vi "i2c_mux_demux.vi"() -> ()   [LabVIEW 2014]
uses:
  mux_state.ctl
  demux_state.ctl
  Common/fractional_phase.ctl
  <vilib>/Platform/TimedLoop/XDataNode/timing_clust.ctl
  <vilib>/Platform/TimedLoop/XDataNode/nitl_modes.ctl
  <vilib>/Platform/TimedLoop/XDataNode/wakeup.ctl
  Common/i2c_status.ctl
  Common/demux_command.ctl
  Common/i2c_command.ctl
  <vilib>/rvi/Emulation/niFpgaGetClockAttributes.vi
  <vilib>/rvi/Emulation/niFpgaSctlEmulationGetInTimedLoop.vi
  <vilib>/rvi/Emulation/niFpgaEmulationReportErrorSimple.vi
  <vilib>/rvi/DataTransferAndStorage/Container/Common/niFpgaContainerExecOnDevCompGetState.vi
  <vilib>/rvi/Emulation/niFpgaEmulationIsFPGAContextNoSignature.vi
  <vilib>/rvi/errors/niFpgaSetErrorForExecOnDevCompSimple.vi
  <vilib>/rvi/eio/common/nirviEmuReportErrorAndStop.vi
  <vilib>/rvi/DataTransferAndStorage/Container/Common/niFpgaContainerGetUniqueNameForEmu.vi
  <vilib>/rvi/FIFO/Fifo_Resource/nirvififoEmulationSetSize.vi
  <vilib>/rvi/FIFO/Fifo_Resource/nirviFifoEmulationQueueMgr.vi
  <instcachedir>/0/nirviFifoEmulationQueueMgr_E5CAEC123FF24DC58D834DCA3CDAA9B5.lvgen/nirviFifoEmulationQueueMgr_E5CAEC123FF24DC58D834DCA3CDAA9B5_002.vi
  <vilib>/rvi/FIFO/Fifo_Resource/nirvififoEmulationDetermineInputValidOut.vi
  <vilib>/rvi/FIFO/Fifo_Resource/nirvififoEmulationCreateLock.vi
  <vilib>/rvi/Emulation/niFpgaProcessEmulError.vi
  <vilib>/rvi/FIFO/Fifo_Resource/nirvififoEmulationObtainLock.vi
  <vilib>/rvi/FIFO/Fifo_Resource/nirvififoEmulationReleaseLock.vi
  <vilib>/rvi/occurrence/nirviWaitOnOccurrenceBase.vi
  <vilib>/rvi/errors/nirviReportUnexpectedCaseInternalError.vi
  <vilib>/rvi/errors/nirviReportUnexpectedCaseInternalError (U32).vi
  <vilib>/Utility/error.llb/Clear Errors.vi
  <vilib>/rvi/interface/RandomDataEmulation/niFpgaRandomDataHandleErrors.vi
  <vilib>/rvi/Emulation/niFpgaCriticalErrorInLSC.vi
  <instcachedir>/0/nirviFifoEmulationQueueMgr_E5CAEC123FF24DC58D834DCA3CDAA9B5.lvgen/nirviFifoEmulationQueueMgr_E5CAEC123FF24DC58D834DCA3CDAA9B5_001.vi
  <vilib>/rvi/eio/common/nirviEmuTemplateMethod_errors.vi
  <vilib>/rvi/DataTransferAndStorage/Container/XNode/niFpgaContainer.xnode
  <vilib>/rvi/FIFO/Fifo_Resource/niFpgaFifoEmulationRefIn.vi
  <vilib>/Platform/TimedLoop/XDataNode/XDataNode.xnode
  <vilib>/eio/EIONode/EIONode.xnode
  <vilib>/Platform/TimedLoop/XDataNode/XDNodeRunTimeDep.lvlib
  fpga_globals.vi
panel:
  in  "Lo rate half period":u16
  out "FPGA code version":i16
  in  "ASAP timer phase advance":T1[](array[typedef])=[0.0, 0.0, 0.0, 0.0, 0.0, 0.0]
  out "Sequence num":u8
  in  "Command hard trigger":bool=TRUE
  in  "Output enable":bool[](array[boolean])=[FALSE, FALSE, FALSE, FALSE, FALSE, FALSE]
  out "Drain count":u8
  out "Hard trigger mode":bool
  out "Drain FIFO":bool
  out "Demux data":u8
  out "Demux  Read inhibit":bool
  out "Hardware trigger enable":bool
  in  "Finder":bool
  in  "ASAP timer initial phase":T1[](array[typedef])=[0.0, 0.0, 0.0, 0.0, 0.0, 0.0]
  out "Timestamp":u16
  out "Trigger wait":bool
  out "Local FIFO full":bool
  out "Demux bus number":fxp<+,8,8>
  out "Demux data ready":bool
  out "Demux state":T2
  out "Mux bus number":fxp<+,3,3>
  out "Host FIFO full":bool
  out "Mux Read inhibit":bool
  out "Mux data ready":bool
  out "Mux data":u8
  out "Mux state":T3
  in  "I2C clock divisor":u8=25
  # "Current timestamp\nfor I2C status notifications."
  # "ASAP finder switch"
  # "The phase in radians is pi times this number. See phase_timer_out.vi for details"
  # "Enable timer outputs"
  # "If true, command operation uses hard trigger mode,\notherwise soft trigger."
  # "Locals:"
  # "Debugging:"
  # "Command sequence number, from host command FIFO"
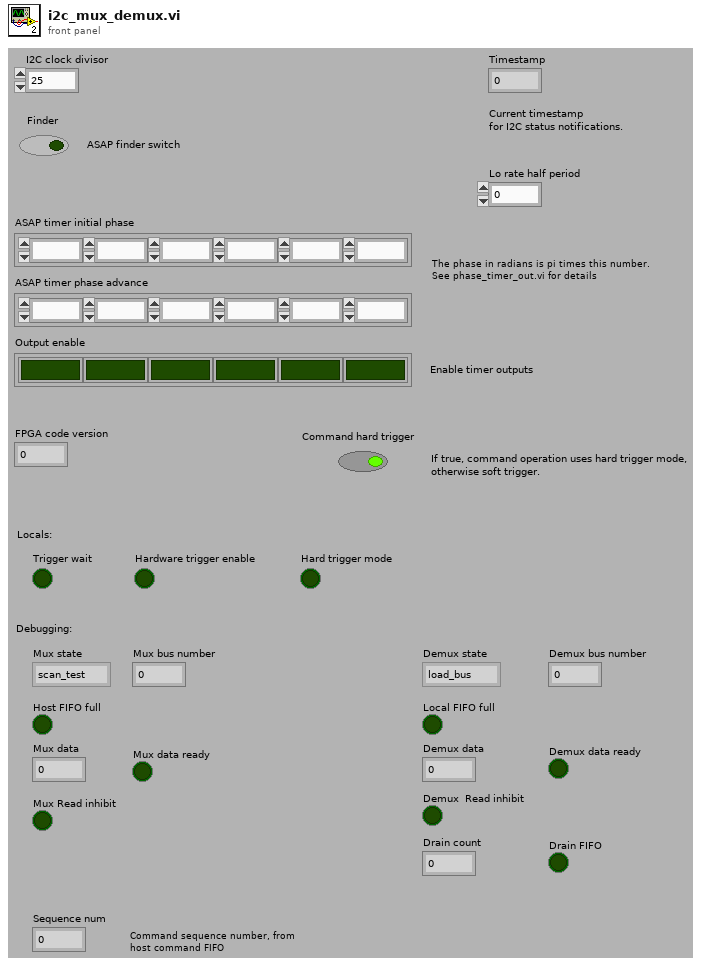
[diagram p1: front panel]
types:
  T1 = typedef "fractional_phase.ctl" = fxp<+,32,1>
  T2 = typedef "demux_state.ctl" = enum8{"load_bus", "load_count", "copying", "wait_trigger"}
  T3 = typedef "mux_state.ctl" = enum8{"scan_test", "push_bus", "push_TS_hi", "push_TS_lo", "copy_code", "load_arg", "copy_arg", "load_count", "copy_data"}
  T4 = typedef "XDNodeRunTimeDep.lvlib/timing_clust.ctl" = cluster{"Expected End [f-1]":u64, "Actual End [f-1]":u64, "Finished Late? [f-1]":bool, "Expected End [i-1]":u64, "Actual End [i-1]":u64, "Finished Late? [i-1]":bool, "Expected Start [i]":u64, "Actual Start [i]":u64, "Expected Start [f]":u64, "Actual Start [f]":u64, "Source Name":string, "Structure Name":string, "Period":i64, "Deadline":i64, "Offset":i64, "Start":i64, "Priority":i32, "Timeout":i32, "Mode":T5, "Wakeup Reason":T6, "Error":errorcluster, "Source Type":string, "Secondary Source Type":string, "Global End Time":u64, "Global Start Time":u64, "Frame Duration":u64, "Iteration Duration":u64, "Assigned CPU":i32, "I/O Scan Engine Mode":u32}
  T5 = typedef "XDNodeRunTimeDep.lvlib/nitl_modes.ctl" = enum32{"No Change", "Process missed periods, maintain original phase", "Discard missed periods, maintain original phase", "Process missed periods, ignore original phase", "Discard missed periods, ignore original phase"}
  T6 = typedef "XDNodeRunTimeDep.lvlib/wakeup.ctl" = enum32{"Normal", "Aborted", "Asynchronous wakeup", "Timing source error", "Timed loop error", "Timeout"}
  T7 = typedef "i2c_status.ctl" = enum8{"Invalid", "Command", "I2C start", "Trigger wait", "TX data wait", "Sequence", "Receive data", "I2C error", "Address NACK", "Data NACK", "SDA stuck", "SCL stuck", "Bad command"}
  T8 = typedef "demux_command.ctl" = enum8{"bus_0", "bus_1", "bus_2", "invalid_3", "invalid_4", "drain_fifo", "wait_hard_trigger", "wait_soft_trigger", "trigger_enable"}
  T9 = typedef "i2c_command.ctl" = enum8{"invalid", "start_write", "start_read", "stop", "sequence"}
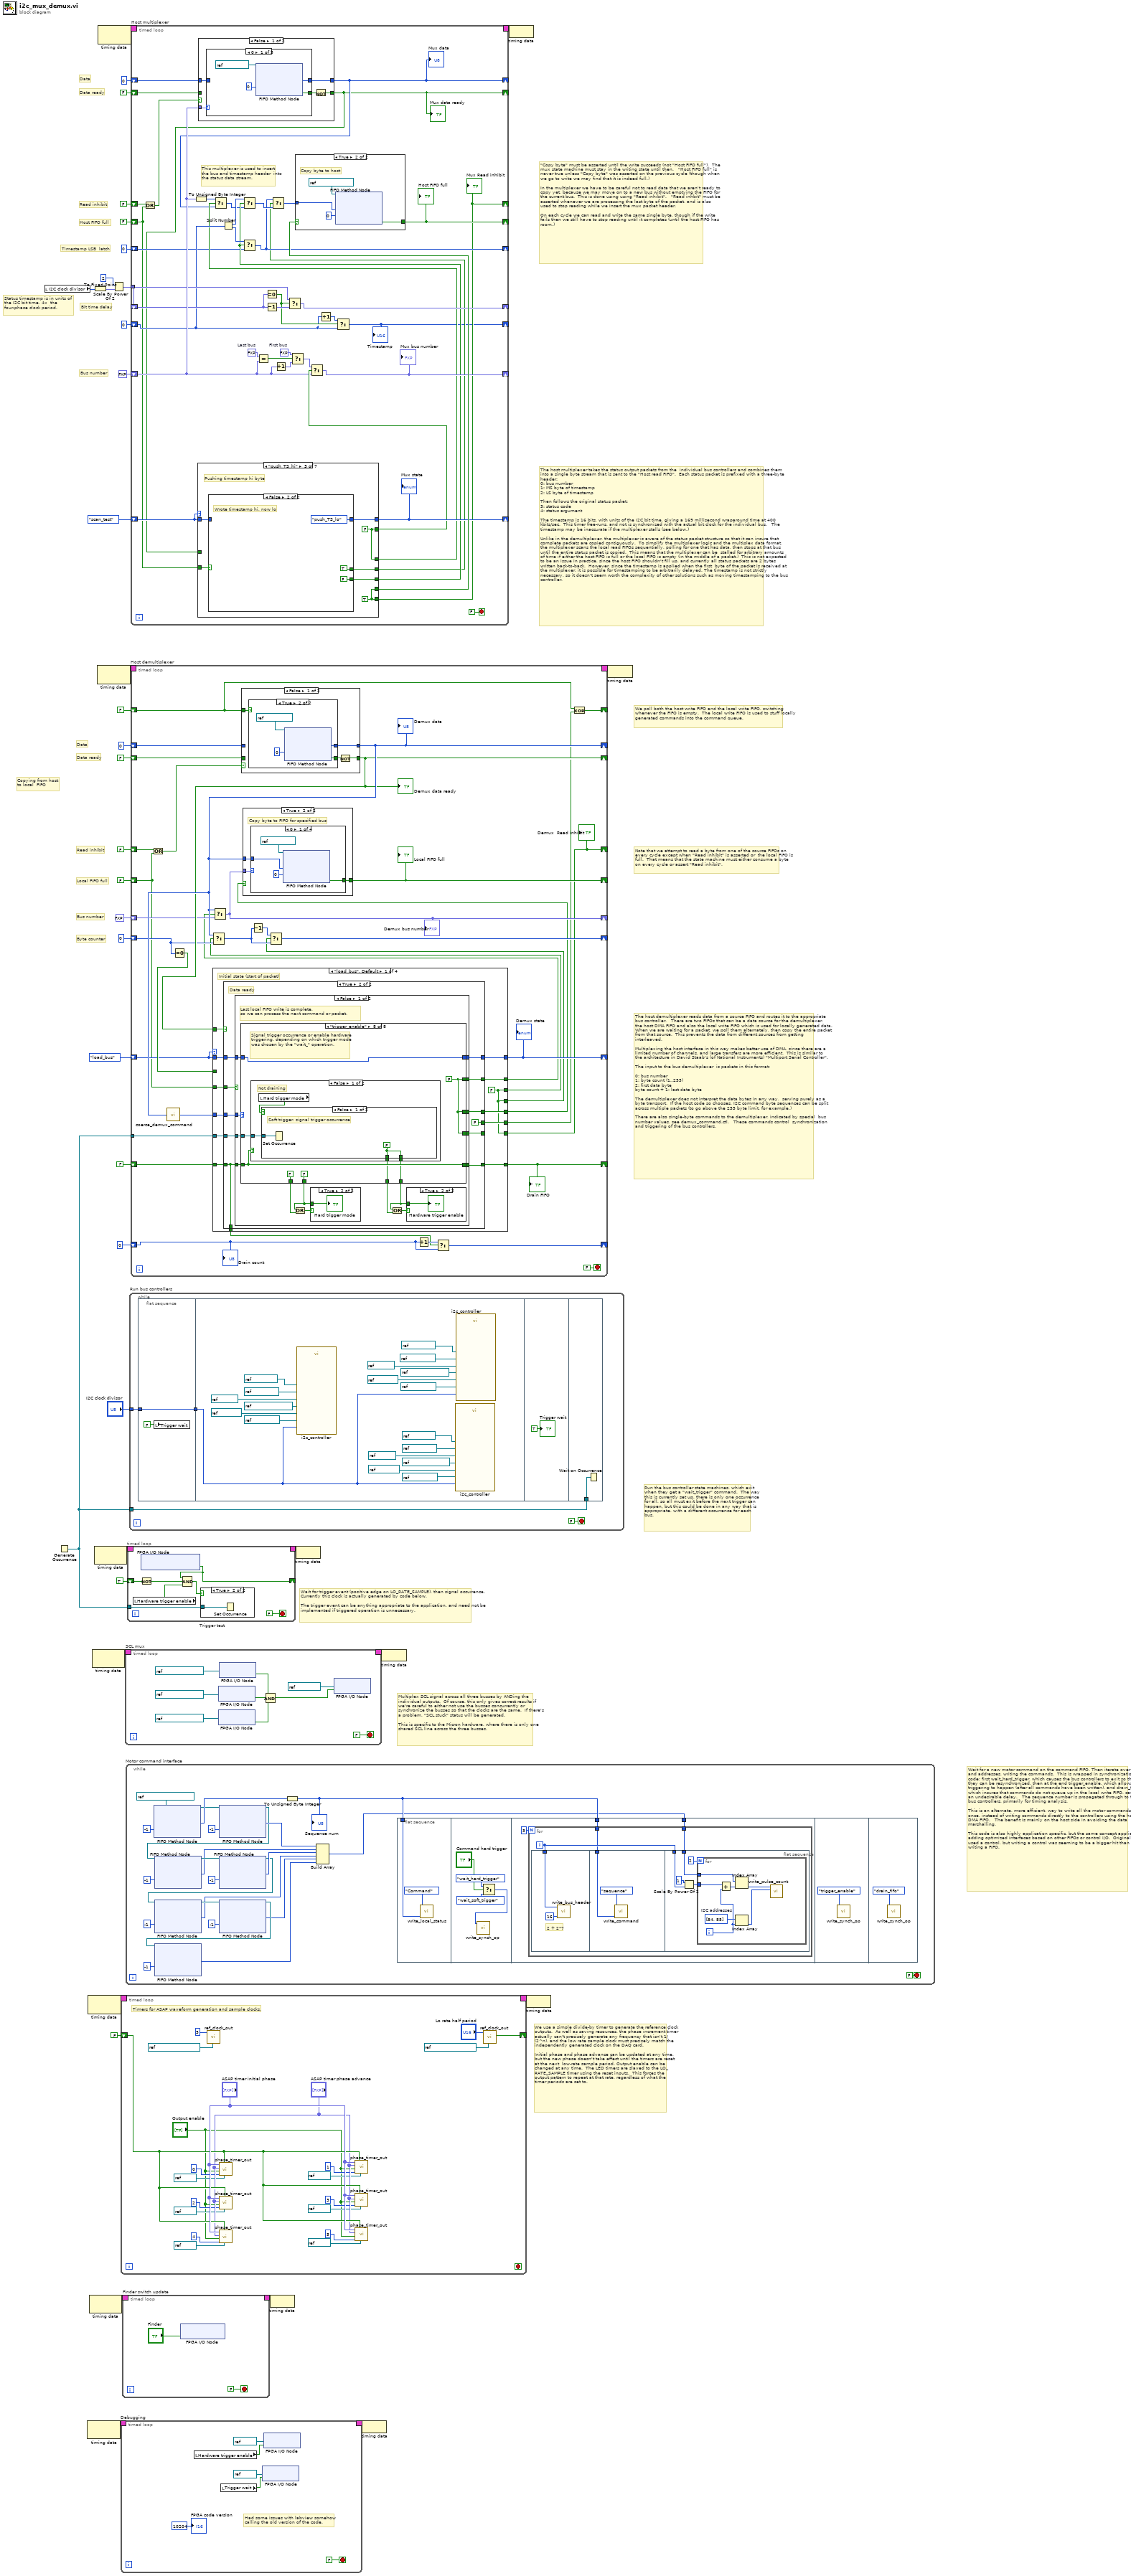
[diagram p0: block diagram]
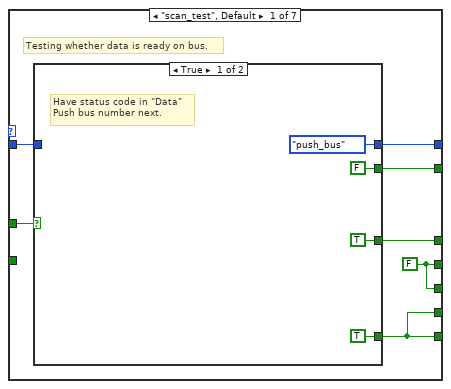
[diagram p3: hidden frame]
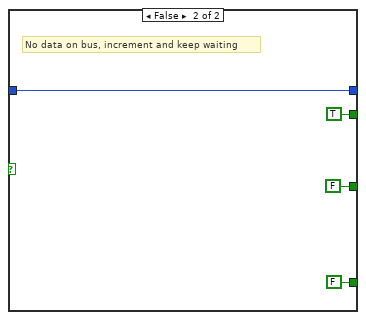
[diagram p4: hidden frame]
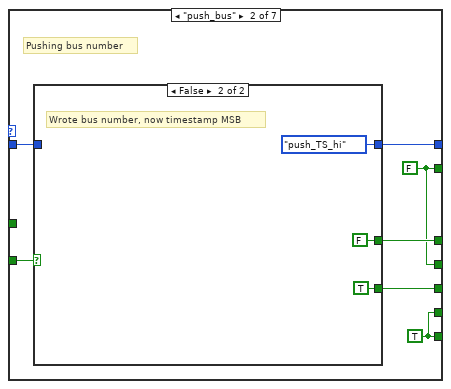
[diagram p5: hidden frame]
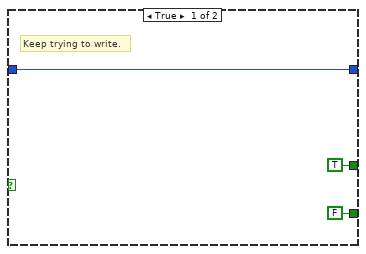
[diagram p6: hidden frame]
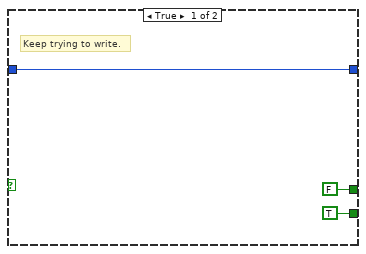
[diagram p7: hidden frame]
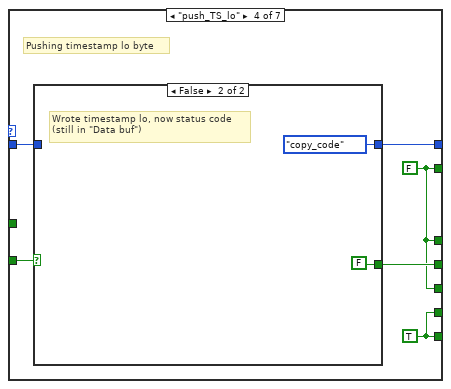
[diagram p8: hidden frame]
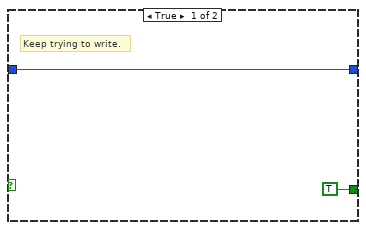
[diagram p9: hidden frame]
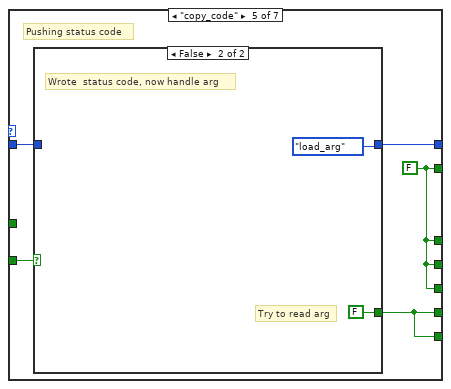
[diagram p10: hidden frame]
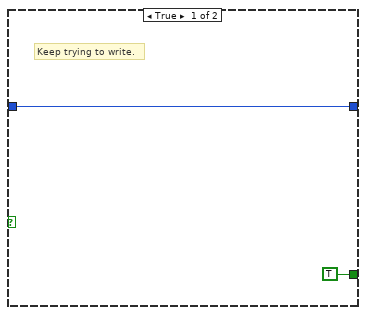
[diagram p11: hidden frame]
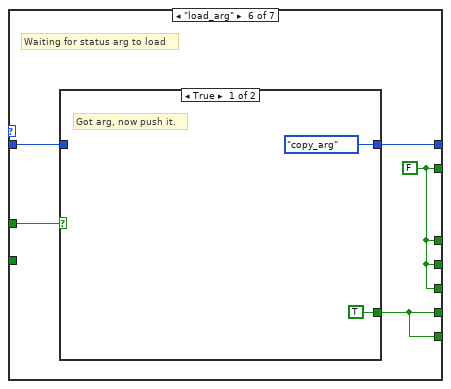
[diagram p12: hidden frame]
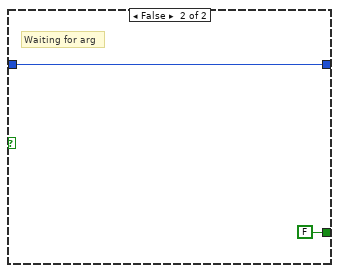
[diagram p13: hidden frame]
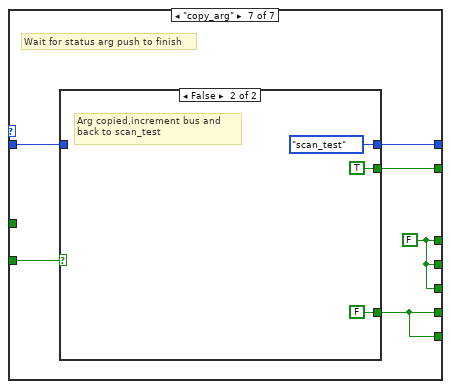
[diagram p14: hidden frame]
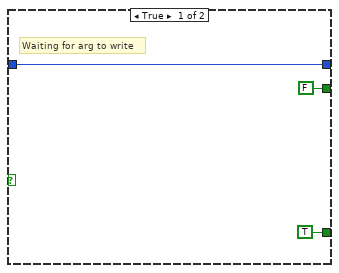
[diagram p15: hidden frame]
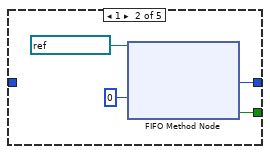
[diagram p16: hidden frame]
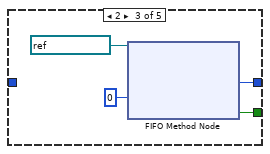
[diagram p17: hidden frame]
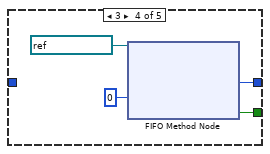
[diagram p18: hidden frame]
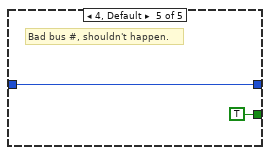
[diagram p19: hidden frame]
diagram:
  # "We use a simple divide-by timer to generate the reference clock outputs.  As well as saving resources, the phase increment timer actually can't precisely generate any frequency that isn't 1/(2^n), and the low rate sample clock must precisely match the independently generated clock on the DAQ card.\n\nInitial phase and phase advance can be updated at any time, but the new phase doesn't take effect until the timers are reset at the next  low-rate sample period. Output enable can be changed at any time.  The LED timers are slaved to the LO_RATE_SAMPLE timer using the reset inputs.  This forces the output pattern to repeat at that rate, regardless of what the timer periods are set to."
  # "Read inhibit"
  # "We poll both the host write FIFO and the local write FIFO, switching whenever the FIFO is empty.  The local write FIFO is used to stuff locally generated commands into the command queue."
  # "Multiplex SCL signal across all three busses by ANDing the individual outputs.  Of course, this only gives correct results if we're careful to either not use the busses concurrently or synchronize the busses so that the clocks are the same.  If there's a problem, \"SCL stuck\" status will be generated.\n\nThis is specific to the Micron hardware, where there is only one shared SCL line across the three busses."
  # "Wait for a new motor command on the command FIFO. Then iterate over buses and addresses, writing the commands.  This is wrapped in synchronization code: first wait_hard_trigger, which causes the bus controllers to exit so that they can be resynchronized, then at the end trigger_enable, which allows triggering to happen (after all commands have been written), and drain_fifo, which insures that commands do not queue up in the local write FIFO, causing an undesirable delay.   The sequence number is propagated through to the bus controllers, primarily for timing analysis.\n\nThis is an alternate, more efficient, way to write all the motor commands at once, instead of writing commands directly to the controllers using the host DMA FIFO.   The benefit is mainly on the host side in avoiding the data marshalling.\n\nThis code is also highly application specific, but the same concept applies of adding optimized interfaces based on other FIFOs or control I/O.  Originally this used a control, but writing a control was seeming to be a bigger hit than writing a FIFO."
  # "Run the bus controller state machines, which exit when they get a \"wait_trigger\" command.  The way this is currently set up, there is only one occurrence for all, so all must exit before the next trigger can happen, but this could be done in any way that is appropriate, with a different occurrence for each bus."
  # "Wait for trigger event (positive edge on LO_RATE_SAMPLE), then signal occurrence.  Currently this clock is actually generated by code below.\n\nThe trigger event can be anything appropriate to the application, and need not be implemented if triggered operation is unnecessary."
  # "\"Copy byte\" must be asserted until the write succeeds (not \"Host FIFO full\").  The mux state machine must stay in the writing state until then.   \"Host FIFO full\" is never true unless \"Copy byte\" was asserted on the previous cycle (though when we go to write we may find that it is indeed full.)\n\nIn the multiplexer we have to be careful not to read data that we aren't ready to copy yet, because we may move on to a new bus without emptying the FIFO for the current bus.  This is done using using \"Read inhibit\".   \"Read inhbit\" must be asserted whenever we are processing the last byte of the packet, and is also used to stop reading while we insert the mux packet header. \n\nOn each cycle we can read and write the same single byte, though if the write fails then we still have to stop reading until it completes (until the host FIFO has room.)"
  # "Read inhibit"
  # "Timestamp LSB  latch"
  # "The host multiplexer takes the status output packets from the  individual bus controllers and combines them into a single byte stream that is sent to the \"Host read FIFO\".  Each status packet is prefixed with a three-byte header:\n0: bus number\n1: MS byte of timestamp\n2: LS byte of timestamp\n\nThen follows the original status packet:\n3: status code\n4: status argument \n\nThe timestamp is 16 bits, with units of the I2C bit time, giving a 169 millisecond wraparound time at 400 kbits/sec.  This timer free-runs, and not is synchronized with the actual bit clock for the individual bus.   The timestamp may be inaccurate if the multiplexer stalls (see below.)\n\nUnlike in the demultiplexer, the multiplexer is aware of the status packet structure so that it can insure that complete packets are copied contiguously.  To simplify the multiplexer logic and the multiplex data format, the multiplexer scans the local read FIFOs sequentially, polling for one that has data, then stops at that bus until the entire status packet is copied.  This means that the multiplexer can be  stalled for arbitrary amounts of time if either the host FIFO is full or the local FIFO is empty (in the middle of a packet.)  This is not expected to be an issue in practice, since the host FIFO shouldn't fill up, and currently all status packets are 2 bytes written back-to-back.  However, since the timestamp is applied when the first  byte of the packet is received at the multiplexer, it is possible for timestamping to be arbitrarily delayed. The timestamp is not strictly necessary, so it doesn't seem worth the complexity of other solutions such as moving timestamping to the bus controller."
  # "Status timestamp is in units of the I2C bit time, 4x  the four-phase clock period."
  # "Bit time delay"
  # "Bus number"
  # "Host FIFO full"
  # "Data"
  # "Data ready"
  # "Byte counter"
  # "Bus number"
  # "Local FIFO full"
  # "Copying from host to local  FIFO"
  # "Data"
  # "Data ready"
  # "The host demultiplexer reads data from a source FIFO and routes it to the appropriate bus controller.   There are two FIFOs that can be a data source for the demultiplexer, the host DMA FIFO and also the local write FIFO which is used for locally generated data.   When we are waiting for a packet, we poll them alternately, then copy the entire packet from that source.  This prevents the data from different sources from getting interleaved.\n\nMultiplexing the host interface in this way makes better use of DMA, since there are a limited number of channels, and large transfers are more efficient.  This is similar to the architecture in David Staab's (of National Instruments) \"Multiport Serial Controller\".\n\nThe input to the bus demultiplexer  is packets in this format:\n\n0: bus number\n1: byte count (1..255)\n2: first data byte\nbyte count + 1: last data byte\n\nThe demultiplexer does not interpret the data bytes in any way,  serving purely as a byte transport.  If the host code so chooses, I2C command byte sequences can be split across multiple packets (to go above the 255 byte limit, for example.)\n\nThere are also single-byte commands to the demultiplexer, indicated by special  bus number values, see demux_command.ctl.   These commands control  synchronization and triggering of the bus controllers."
  # "Note that we attempt to read a byte from one of the source FIFOs on every cycle except when \"Read inhibit\" is asserted or  the local FIFO is full.  That means that the state machine must either consume a byte on every cycle or assert \"Read inhibit\"."
  n1 = local read "I2C clock divisor"() -> (w23:u8)
  n2 = Generate Occurrence() -> (w8:refnum<k4>)
  n3 = node-c288() -> (w5:T4)  [unwired: 1 in]
  n4 = node-c288() -> (w3:T4)  [unwired: 1 in]
  n5 = node-c288() -> (w14:T4)  [unwired: 1 in]
  n6 = node-c288() -> (w12:T4)  [unwired: 1 in]
  n7 = To Fixed-Point(number=w23) -> (fixed-point=w24:fxp<+,10,10>)  [unwired: 1 in]
  n8 = node-c288() -> (w18:T4)  [unwired: 1 in]
  n9 = node-c288() -> (w39:T4)  [unwired: 1 in]
  n10 = node-c288() -> (w32:T4)  [unwired: 1 in]
  n11 = Scale By Power Of 2(n=2, x=w24) -> (x*2^n=w25:fxp<+,10,10>)
  n12 = timed-loop "Debugging" {
    timing: w5 -> [_]
    timing-out: [_] -> w4
    stop <- FALSE stop-if-true
    # "Had some issues with labview somehow\ncalling the old version of the code."
    n13 = local read "Hardware trigger enable"() -> (w44:bool)
    n14 = local read "Trigger wait"() -> (w43:bool)
    n15 = xnode "FPGA I/O Node"("I/O Item"=w43, "FPGA I/O In"=refnum<k21> "LED9" ("FPGA I/O")) -> ()  [unwired: 1 out]
    n16 = xnode "FPGA I/O Node"("I/O Item"=w44, "FPGA I/O In"=refnum<k21> "LED8" ("FPGA I/O")) -> ()  [unwired: 1 out]
    "FPGA code version" <- i16 10204
  }
  n17 = timed-loop {
    timing: w3 -> [_]
    timing-out: [_] -> w2
    shift-right: [w66] -> _
    shift-left: FALSE ("Pos edge") -> [w68]
    stop <- _ stop-if-true
    # "Timers for ASAP waveform generation and sample clocks."
    n18 = call "ref_clock_out.vi"("FPGA I/O"=refnum<k21> "FPGA_10MHZ_REF", "Half period"=u16 5) -> ()  [unwired: 9 in, 1 out]
    n19 = call "phase_timer_out.vi"("FPGA I/O"=refnum<k21> "LED0", "Reset"=w68, "Channel number"=u8 0, "Output enable"="Output enable", "Phase advance"="ASAP timer phase advance", "Initial phase"="ASAP timer initial phase") -> ()  [unwired: 5 in, 1 out]
    n20 = call "phase_timer_out.vi"("FPGA I/O"=refnum<k21> "LED2", "Reset"=w68, "Channel number"=u8 2, "Output enable"="Output enable", "Phase advance"="ASAP timer phase advance", "Initial phase"="ASAP timer initial phase") -> ()  [unwired: 5 in, 1 out]
    n21 = call "phase_timer_out.vi"("FPGA I/O"=refnum<k21> "LED4", "Reset"=w68, "Channel number"=u8 4, "Output enable"="Output enable", "Phase advance"="ASAP timer phase advance", "Initial phase"="ASAP timer initial phase") -> ()  [unwired: 5 in, 1 out]
    n22 = call "phase_timer_out.vi"("FPGA I/O"=refnum<k21> "LED1", "Reset"=w68, "Channel number"=u8 1, "Output enable"="Output enable", "Phase advance"="ASAP timer phase advance", "Initial phase"="ASAP timer initial phase") -> ()  [unwired: 5 in, 1 out]
    n23 = call "phase_timer_out.vi"("FPGA I/O"=refnum<k21> "LED3", "Reset"=w68, "Channel number"=u8 3, "Output enable"="Output enable", "Phase advance"="ASAP timer phase advance", "Initial phase"="ASAP timer initial phase") -> ()  [unwired: 5 in, 1 out]
    n24 = call "phase_timer_out.vi"("FPGA I/O"=refnum<k21> "LED5", "Reset"=w68, "Channel number"=u8 5, "Output enable"="Output enable", "Phase advance"="ASAP timer phase advance", "Initial phase"="ASAP timer initial phase") -> ()  [unwired: 5 in, 1 out]
    n25 = call "ref_clock_out.vi"("FPGA I/O"=refnum<k21> "LO_RATE_SAMPLE", "Half period"="Lo rate half period") -> ("Pos edge"=w66:bool)  [unwired: 9 in]
  }
  n26 = timed-loop "Finder switch update" {
    timing: w14 -> [_]
    timing-out: [_] -> w13
    stop <- FALSE stop-if-true
    n27 = xnode "FPGA I/O Node"("FINDER_ON"="Finder") -> ()  [unwired: 1 in, 1 out]
  }
  n28 = timed-loop "SCL mux" {
    timing: w12 -> [_]
    timing-out: [_] -> w11
    stop <- FALSE stop-if-true
    n29 = xnode "FPGA I/O Node"("FPGA I/O In"=refnum<k21> "SCL_OUT1_DUM" ("SCL pin")) -> ("I/O Item"=w80:bool)  [unwired: 1 out]
    n30 = xnode "FPGA I/O Node"("FPGA I/O In"=refnum<k21> "SCL_OUT2_DUM" ("SDA pin")) -> ("I/O Item"=w79:bool)  [unwired: 1 out]
    n31 = xnode "FPGA I/O Node"("FPGA I/O In"=refnum<k21> "SCL_OUT0_DUM" ("SCL pin")) -> ("I/O Item"=w81:bool)  [unwired: 1 out]
    n32 = Compound Arithmetic op=AND(w81, w80, w79) -> (w77:bool)
    n33 = xnode "FPGA I/O Node"("I/O Item"=w77, "FPGA I/O In"=refnum<k21> "SCL_OUT" ("SCL pin")) -> ()  [unwired: 1 out]
  }
  n34 = while "Motor command interface" {
    stop <- FALSE stop-if-true
    n35 = xnode ("FIFO Method Node")("Timeout"=-1, "FIFO In"=refnum<k21> "Host command FIFO") -> ("Element"=w106:i16, "FIFO Out"=w104:refnum<k21>)  [unwired: 1 out]
    n36 = xnode ("FIFO Method Node")("Timeout"=-1, "FIFO In"=w104) -> ("Element"=w102:i16, "FIFO Out"=w101:refnum<k21>)  [unwired: 1 out]
    n37 = xnode ("FIFO Method Node")("Timeout"=-1, "FIFO In"=w101) -> ("Element"=w92:i16, "FIFO Out"=w99:refnum<k21>)  [unwired: 1 out]
    n38 = xnode ("FIFO Method Node")("Timeout"=-1, "FIFO In"=w99) -> ("Element"=w91:i16, "FIFO Out"=w87:refnum<k21>)  [unwired: 1 out]
    n39 = xnode ("FIFO Method Node")("Timeout"=-1, "FIFO In"=w87) -> ("Element"=w90:i16, "FIFO Out"=w96:refnum<k21>)  [unwired: 1 out]
    n40 = xnode ("FIFO Method Node")("Timeout"=-1, "FIFO In"=w96) -> ("Element"=w89:i16, "FIFO Out"=w94:refnum<k21>)  [unwired: 1 out]
    n41 = xnode ("FIFO Method Node")("Timeout"=-1, "FIFO In"=w94) -> ("Element"=w88:i16)  [unwired: 2 out]
    n42 = To Unsigned Byte Integer(number=w106) -> (unsigned 8bit integer=w109:u8)
    "Sequence num" <- w109
    n43 = Build Array(w102, w92, w91, w90, w89, w88) -> (w105:i16[])
    n44 = flat-sequence {
      tunnel: w109 -> [w111]
      tunnel: w105 -> [w118]
      tunnel: w109 -> [w117]
      frame #0 {
        n45 = call "write_local_status.vi"("Argument"=w111, "Status code"=i2c_status."Command") -> ()  [unwired: 10 in]
      }
      frame #1 {
        n46 = Select(t=demux_command."wait_hard_trigger" ("Bus"), s="Command hard trigger", f=demux_command."wait_soft_trigger" ("Bus")) -> (s? t:f=w113:T8)
        n47 = call "write_synch_op.vi"("Bus"=w113) -> ()  [unwired: 11 in]
      }
      frame #2 {
        n48 = for {
          N: 3 -> [_]
          tunnel: w117 -> [w120]
          tunnel: w118 -> [w121]
          i -> [w122]
          n49 = flat-sequence {
            tunnel: w122 -> [w123]
            tunnel: w120 -> [w125]
            tunnel: w121 -> [w128]
            tunnel: w122 -> [w129]
            frame #0 {
              # "2 + 2*7"
              n50 = call "write_bus_header.vi"("Count"=u8 16, "Bus"=w123) -> ()  [unwired: 10 in]
            }
            frame #1 {
              n51 = call "write_command.vi"("Arg"=w125, "Command"=i2c_command."sequence") -> ()  [unwired: 10 in]
            }
            frame #2 {
              n52 = Scale By Power Of 2(n=1, x=w129) -> (x*2^n=w130:i32)
              n53 = for {
                N: 2 -> [_]
                tunnel: w130 -> [w135]
                tunnel: w128 -> [w133]
                i -> [w134]
                w138 = u8[] [84, 85]  # I2C addresses
                n54 = Add(x=w135, y=w134) -> (x+y=w136:i32)
                n55 = Index Array(array=w133, index=w136) -> (element=w132:i16)
                n56 = Index Array(array=w138, index=w134) -> (element=w137:u8)
                n57 = call "write_pulse_count.vi"("Address"=w137, "Pulse count"=w132) -> ()  [unwired: 10 in]
              }
            }
          }
        }
      }
      frame #3 {
        n58 = call "write_synch_op.vi"("Bus"=demux_command."trigger_enable") -> ()  [unwired: 11 in]
      }
      frame #4 {
        n59 = call "write_synch_op.vi"("Bus"=demux_command."drain_fifo") -> ()  [unwired: 11 in]
      }
    }
  }
  n60 = timed-loop "Trigger test" {
    timing: w18 -> [_]
    timing-out: [_] -> w17
    shift-right: [w146] -> _
    shift-left: TRUE ("RTSI1") -> [w147]
    tunnel: w8 -> [w143]
    stop <- FALSE stop-if-true
    n61 = local read "Hardware trigger enable"() -> (w141:bool)
    n62 = Not(x=w147) -> (.not. x?=w145:bool)
    n63 = xnode "FPGA I/O Node"() -> ("LO_RATE_SAMPLE"=w146:bool)  [unwired: 1 in, 1 out]
    n64 = Compound Arithmetic op=AND(w146, w145, w141) -> (w144:bool)
    n65 = case shown="True" w144 {
      tunnel: w143 -> [_ w148]
      frame False {
      }
      frame True {
        n66 = Set Occurrence(w148) -> ()
      }
    }
  }
  n67 = while "Run bus controllers" {
    tunnel: "I2C clock divisor" -> [w154]
    tunnel: w8 -> [w152]
    stop <- FALSE stop-if-true
    n68 = flat-sequence {
      tunnel: w154 -> [w156]
      tunnel: [w156] -> w151
      tunnel: w151 -> [w173]
      tunnel: w152 -> [w177]
      frame #0 {
        n69 = local write "Trigger wait"(FALSE ("Trigger wait")) -> ()
      }
      frame #1 {
        n70 = call "i2c_controller.vi"("SDA in pin"=refnum<k21> "SDA_IN0" ("SDA pin"), "I2C clock divisor"=w173, "SCL out pin"=refnum<k21> "SCL_OUT0_DUM" ("SCL pin"), "Read FIFO"=refnum<k21> "I2C read 0", "Write FIFO"=refnum<k21> "I2C write 0", "SDA out pin"=refnum<k21> "SDA_OUT0" ("SDA pin"), "SCL in pin"=refnum<k21> "SCL_IN" ("SCL pin")) -> ()  [unwired: 5 in]
        n71 = call "i2c_controller.vi"("SDA in pin"=refnum<k21> "SDA_IN2" ("SDA pin"), "I2C clock divisor"=w173, "SCL out pin"=refnum<k21> "SCL_OUT2_DUM" ("SCL pin"), "Read FIFO"=refnum<k21> "I2C read 2", "Write FIFO"=refnum<k21> "I2C write 2", "SDA out pin"=refnum<k21> "SDA_OUT2" ("SDA pin"), "SCL in pin"=refnum<k21> "SCL_IN" ("SCL pin")) -> ()  [unwired: 5 in]
        n72 = call "i2c_controller.vi"("SDA in pin"=refnum<k21> "SDA_IN1" ("SDA pin"), "I2C clock divisor"=w173, "SCL out pin"=refnum<k21> "SCL_OUT1_DUM" ("SCL pin"), "Read FIFO"=refnum<k21> "I2C read 1", "Write FIFO"=refnum<k21> "I2C write 1", "SDA out pin"=refnum<k21> "SDA_OUT1" ("SDA pin"), "SCL in pin"=refnum<k21> "SCL_IN" ("SCL pin")) -> ()  [unwired: 5 in]
      }
      frame #2 {
        "Trigger wait" <- TRUE ("Trigger wait")
      }
      frame #3 {
        n73 = Wait on Occurrence(2:w177) -> ()  [unwired: 2 in, 1 out]
      }
    }
  }
  n74 = timed-loop "Host demultiplexer" {
    timing: w39 -> [_]
    timing-out: [_] -> w38
    shift-right: [w208] -> _
    shift-left: FALSE ("Timed Out?") -> [w192]
    shift-right: [w210] -> _
    shift-left: FALSE -> [w189]
    shift-right: [w211] -> _
    shift-left: u8 0 ("Element") -> [w206]
    shift-right: [w202] -> _
    shift-left: u8 0 ("Timeout") -> [w203]
    shift-right: [w209] -> _
    shift-left: demux_state."load_bus" ("Demux state") -> [w194]
    shift-right: [w199] -> _
    shift-left: fxp<+,2,2> 0.0 ("Timeout") -> [w200]
    shift-right: [w187] -> _
    shift-left: FALSE -> [w188]
    shift-right: [w191] -> _
    shift-left: FALSE -> [w193]
    tunnel: w8 -> [w184]
    shift-right: [w183] -> _
    shift-left: FALSE ("Hardware trigger enable") -> [w182]
    shift-right: [w179] -> _
    shift-left: u8 0 ("Timeout") -> [w180]
    stop <- FALSE stop-if-true
    n75 = Or(x=w193, y=w192) -> (x .or. y?=w190:bool)
    n76 = Equal To 0?(x=w203) -> (x = 0?=w201:bool)
    n77 = case shown="False" w190 {
      tunnel: [w406 w416] -> w211
      tunnel: [w405 w415] -> w210
      tunnel: w206 -> [_ w416]
      tunnel: w188 -> [w403 _]
      tunnel: w189 -> [_ w415]
      frame False {
        n78 = case shown="True" w403 {
          tunnel: [w408 w412] -> w406
          tunnel: [w407 w411] -> w404
          frame False {
            n79 = xnode ("FIFO Method Node")("Timeout"=0, "FIFO In"=refnum<k21> "Host write FIFO") -> ("Element"=w408:u8, "Timed Out?"=w407:bool)  [unwired: 1 out]
          }
          frame True {
            n80 = xnode ("FIFO Method Node")("Timeout"=0, "FIFO In"=refnum<k21> "Local write") -> ("Element"=w412:u8, "Timed Out?"=w411:bool)  [unwired: 1 out]
          }
        }
        n81 = Not(x=w404) -> (.not. x?=w405:bool)
      }
      frame True {
        # "Hold off reading on this cycle. \nData remains unchanged."
      }
    }
    "Demux data ready" <- w210
    "Demux data" <- w211
    n82 = call "coerce_demux_command.vi"("U8 code"=w211) -> ("Demux command"=w185:T8)
    n83 = case shown="\"load_bus\", Default" w194 {
      tunnel: [w212 w348 w359 w393] -> w198
      tunnel: [w212 w348 w362 w393] -> w197
      tunnel: [w224 w351 w362 w393] -> w196
      tunnel: [w222 w351 w368 w393] -> w195
      tunnel: [w223 w354 w365 w392] -> w209
      tunnel: w201 -> [_ _ w364 _]
      tunnel: w192 -> [w221 _ w367 _]
      tunnel: w194 -> [w220 w352 w366 w391]
      tunnel: [w212 w351 w362 TRUE ("x = 0?")] -> w191
      tunnel: [w217 w351 w362 w393] -> w186
      tunnel: w210 -> [w219 w353 w363 _]
      tunnel: w185 -> [w218 _ _ _]
      tunnel: w184 -> [w216 _ _ _]
      tunnel: [w215 w349 w360 w390] -> w183
      tunnel: w182 -> [w214 w349 w360 w390]
      tunnel: [w213 w350 w361 FALSE ("Hardware trigger enable")] -> w178
      frame "load_bus", Default {
        w212 = FALSE ("x = 0?")
        # "Initial state (start of packet)"
        n84 = case shown="True" w219 {
          tunnel: [w226 w239] -> w224
          tunnel: [w228 w238] -> w223
          tunnel: [w226 w237] -> w222
          tunnel: w221 -> [_ w236]
          tunnel: w220 -> [w228 w235]
          tunnel: w218 -> [_ w234]
          tunnel: [TRUE ("x = 0?") FALSE ("x = 0?")] -> w217
          tunnel: w216 -> [_ w232]
          tunnel: [w226 w231] -> _
          tunnel: [w226 w230] -> w215
          tunnel: w214 -> [_ w229]
          tunnel: [FALSE ("Hardware trigger enable") w229] -> w213
          frame False {
            w226 = FALSE ("x = 0?")
            # "Data not ready, wait for bus number or command.\nIf we were draining the FIFO, then we're done."
          }
          frame True {
            # "Data ready"
            n85 = case shown="False" w236 {
              tunnel: [w254 FALSE ("x = 0?")] -> w239
              tunnel: [w252 w345] -> w238
              tunnel: [w253 TRUE ("x = 0?")] -> w237
              tunnel: w235 -> [w250 w345]
              tunnel: w234 -> [w251 _]
              tunnel: w232 -> [w249 _]
              tunnel: [w248 FALSE ("Hardware trigger enable")] -> w231
              tunnel: w229 -> [w247 w343]
              tunnel: [w246 w343] -> w230
              frame False {
                # "Last local FIFO write is complete,\nso we can process the next command or packet."
                n86 = case shown="\"trigger_enable\"" w251 {
                  tunnel: [TRUE ("x = 0?") TRUE ("x = 0?") TRUE ("x = 0?") FALSE ("x = 0?") FALSE ("x = 0?") w297 w315 w331] -> w254
                  tunnel: [FALSE ("x = 0?") FALSE ("x = 0?") FALSE ("x = 0?") FALSE ("x = 0?") FALSE ("x = 0?") w297 w315 w331] -> w253
                  tunnel: [demux_state."load_count" ("Demux state") demux_state."load_count" ("Demux state") demux_state."load_count" ("Demux state") w281 w287 w298 w316 w333] -> w252
                  tunnel: w250 -> [_ _ _ w281 w287 w295 w313 w333]
                  tunnel: w249 -> [_ _ _ _ _ _ _ w332]
                  tunnel: [FALSE ("Hardware trigger enable") FALSE ("Hardware trigger enable") FALSE ("Hardware trigger enable") FALSE ("Hardware trigger enable") FALSE ("Hardware trigger enable") w296 w314 w331] -> w248
                  tunnel: w247 -> [w259 w266 w273 _ _ w294 w312 w330]
                  tunnel: [w259 w266 w273 TRUE ("Hardware trigger enable") TRUE ("Hardware trigger enable") w294 w312 w330] -> w246
                  tunnel: [w258 w265 w272 w278 w284 w293 w311 w329] -> w244
                  tunnel: [w258 w265 w272 w278 w284 w292 w310 w328] -> w243
                  tunnel: [w257 w264 w271 w278 w284 w291 w309 FALSE ("Hardware trigger enable")] -> w241
                  tunnel: [w257 w264 w271 w278 w284 w290 w308 FALSE ("Hardware trigger enable")] -> w240
                  frame "bus_0" {
                    w257 = FALSE ("Hardware trigger enable")
                    w258 = FALSE ("Hardware trigger enable")
                  }
                  frame "bus_1" {
                    w264 = FALSE ("Hardware trigger enable")
                    w265 = FALSE ("Hardware trigger enable")
                  }
                  frame "bus_2" {
                    w271 = FALSE ("Hardware trigger enable")
                    w272 = FALSE ("Hardware trigger enable")
                  }
                  frame "invalid_3", Default {
                    w278 = FALSE ("Hardware trigger enable")
                    # "Oops, bad bus number. Drain the FIFO.\nMaybe if we close our eyes it will go away."
                  }
                  frame "drain_fifo" {
                    w284 = FALSE ("Hardware trigger enable")
                    # "Explicit drain of the host FIFO."
                  }
                  frame "wait_soft_trigger" {
                    w297 = FALSE ("x = 0?")
                    n87 = case shown="True" w294 {
                      tunnel: [demux_state."wait_trigger" ("Demux state") w307] -> w298
                      tunnel: [TRUE ("Hardware trigger enable") FALSE ("Hardware trigger enable")] -> w296
                      tunnel: w295 -> [_ w307]
                      tunnel: [FALSE ("Hardware trigger enable") w305] -> w293
                      tunnel: [TRUE ("Hardware trigger enable") w305] -> w292
                      tunnel: [TRUE ("Hardware trigger enable") w305] -> w291
                      tunnel: [FALSE ("Hardware trigger enable") w305] -> w290
                      frame False {
                        # "Clear HTM"
                        # "Hard triggering is disabled immediately."
                        # "Not draining"
                      }
                      frame True {
                        w305 = FALSE ("Hardware trigger enable")
                        # "Draining FIFO, ignore."
                      }
                    }
                  }
                  frame "wait_hard_trigger" {
                    w315 = FALSE ("x = 0?")
                    n88 = case shown="False" w312 {
                      tunnel: [demux_state."wait_trigger" ("Demux state") w325] -> w316
                      tunnel: [TRUE ("Hardware trigger enable") FALSE ("Hardware trigger enable")] -> w314
                      tunnel: w313 -> [_ w325]
                      tunnel: [FALSE ("Hardware trigger enable") w323] -> w311
                      tunnel: [TRUE ("Hardware trigger enable") w323] -> w310
                      tunnel: [FALSE ("Hardware trigger enable") w323] -> w309
                      tunnel: [TRUE ("Hardware trigger enable") w323] -> w308
                      frame False {
                        # "Set HTM"
                        # "Hard triggering is disabled immediately."
                        # "Not draining"
                      }
                      frame True {
                        w323 = FALSE ("Hardware trigger enable")
                        # "Draining FIFO, ignore."
                      }
                    }
                  }
                  frame "trigger_enable" {
                    w331 = FALSE ("Hardware trigger enable")
                    # "Signal trigger occurrence or enable hardware triggering, depending on which trigger mode was chosen by the \"wait_\" operation."
                    n89 = case shown="False" w330 {
                      tunnel: w332 -> [w337 _]
                      tunnel: [w336 w342] -> w329
                      tunnel: [w334 w342] -> w328
                      frame False {
                        # "Not draining"
                        n90 = local read "Hard trigger mode"() -> (w335:bool)
                        n91 = case shown="False" w335 {
                          tunnel: w337 -> [w339 _]
                          tunnel: [w338 TRUE ("Hardware trigger enable")] -> w336
                          tunnel: [w338 FALSE ("Hardware trigger enable")] -> w334
                          frame False {
                            w338 = FALSE ("Hardware trigger enable")
                            # "Soft trigger, signal trigger occurrence"
                            n92 = Set Occurrence(w339) -> ()
                          }
                          frame True {
                            # "Hardware trigger, enable\ntriggering."
                          }
                        }
                      }
                      frame True {
                        w342 = FALSE ("Hardware trigger enable")
                        # "Draining FIFO, so ignore this operation."
                      }
                    }
                  }
                }
                n93 = Or(x=w240, y=w241) -> (x .or. y?=w242:bool)
                n94 = case shown="True" w242 {
                  tunnel: w240 -> [_ w255]
                  frame False {
                  }
                  frame True {
                    "Hard trigger mode" <- w255
                  }
                }
                n95 = Or(x=w244, y=w243) -> (x .or. y?=w245:bool)
                n96 = case shown="True" w245 {
                  tunnel: w244 -> [_ w256]
                  frame False {
                  }
                  frame True {
                    "Hardware trigger enable" <- w256
                  }
                }
              }
              frame True {
                # "If we are still trying to write a full local FIFO, then reading is held off until that situation resolves.   In this case, we just retry the write."
              }
            }
          }
        }
      }
      frame "load_count" {
        w351 = FALSE ("x = 0?")
        # "Loading count byte for packet."
        n97 = case shown="True" w353 {
          tunnel: [FALSE ("x = 0?") TRUE ("x = 0?")] -> w348
          tunnel: [w355 demux_state."copying" ("Demux state")] -> w354
          tunnel: w352 -> [w355 _]
          frame False {
            # "No data yet, wait for count byte"
          }
          frame True {
            # "Data ready"
            # "Have byte count, load and go to next state.  We pre-decrement the count so that  done is true on the last byte.  This means that 0 is not a legal count."
          }
        }
        n98 = And(x=w348, y=w349) -> (x .and. y?=w350:bool)
      }
      frame "copying" {
        w362 = FALSE ("x = 0?")
        # "Copying packet data to local FIFO (or discarding, if draining.)"
        n99 = case shown="True" w363 {
          tunnel: [w369 w377] -> w368
          tunnel: w367 -> [_ w376]
          tunnel: w366 -> [w370 w375]
          tunnel: [w370 w374] -> w365
          tunnel: [w369 w373] -> w359
          tunnel: w364 -> [_ w372]
          tunnel: w360 -> [_ w371]
          frame False {
            w369 = FALSE ("x = 0?")
            # "Though this most likely won't happen as long as data is kept continguous by the FIFO implementation, if we run out of data in the middle of a packet while draining, we keep reading to the end of the packet, even though we have to block.  That way we stop in a good place."
            # "No data, keep waiting"
          }
          frame True {
            # "Data ready"
            n100 = case shown="False" w376 {
              tunnel: [w379 TRUE ("x = 0?")] -> w377
              tunnel: [w381 w386] -> w374
              tunnel: w375 -> [w382 w386]
              tunnel: [TRUE ("x = 0?") FALSE ("x = 0?")] -> w373
              tunnel: w372 -> [w383 _]
              tunnel: w371 -> [w378 _]
              frame False {
                # "If last byte, go back to\ninitial state."
                # "There's data and somewhere to put it.  Decrement count and (attempt) to push the byte.  Or just drop it, if we are draining the FIFO."
                # "FIFO ready"
                n101 = Select(t=demux_state."load_bus" ("Demux state"), s=w383, f=w382) -> (s? t:f=w381:T2)
                n102 = Not(x=w378) -> (.not. x?=w379:bool)
              }
              frame True {
                # "If FIFO full, just wait, asserting \"Copy byte\" to retry\nthe push."
              }
            }
          }
        }
        n103 = And(x=w359, y=w360) -> (x .and. y?=w361:bool)
      }
      frame "wait_trigger" {
        w393 = FALSE ("x = 0?")
        # "This state doesn't\nconsume any data,\nit just waits."
        # "State while waiting for the bus controllers to exit and return back to this VI\nso that they can be restarted in synchrony."
        n104 = case shown="False" w390 {
          tunnel: [w396 demux_state."load_bus" ("Demux state")] -> w392
          tunnel: w391 -> [w395 _]
          frame False {
            # "Not draining."
            n105 = local read "Trigger wait"() -> (w397:bool)
            n106 = case shown="True" w397 {
              tunnel: [w399 demux_state."load_bus" ("Demux state")] -> w396
              tunnel: w395 -> [w399 _]
              tunnel: [TRUE ("I2C Exit on Idle") FALSE ("I2C Exit on Idle")] -> w394
              frame False {
                # "Tell bus controllers to exit as\nsoon as their command queue\nempties out."
                # "Some bus still busy."
              }
              frame True {
                # "If all bus controllers stopped,\ngo back to initial state."
              }
            }
            n107 = global write "fpga_globals.vi" "I2C Exit on Empty"(w394) -> ()
          }
          frame True {
            # "If draining the FIFO, do nothing, just go back to initial state.  Really we shouldn't get in this state if draining."
          }
        }
      }
    }
    "Demux state" <- w209
    "Demux  Read inhibit" <- w191
    "Drain FIFO" <- w183
    n108 = Select(t=w211, s=w197, f=w203) -> (s? t:f=w204:u8)
    n109 = Select(t=w211, s=w196, f=w200) -> (s? t:f=w199:fxp<+,8,8>)
    "Demux bus number" <- w199
    n110 = case shown="True" w195 {
      tunnel: [FALSE ("Timed Out?") w420] -> w208
      tunnel: w211 -> [_ w419]
      tunnel: w199 -> [_ w418]
      frame False {
        # "\"Copy byte\" not asserted"
      }
      frame True {
        # "Copy byte to FIFO for specified bus"
        n111 = case shown="0" w418 {
          tunnel: [w423 w427 w431 FALSE ("Timed Out?")] -> w420
          tunnel: w419 -> [w421 w425 w429 _]
          frame 0 {
            n112 = xnode ("FIFO Method Node")("Element"=w421, "Timeout"=0, "FIFO In"=refnum<k21> "I2C write 0" ("FIFO")) -> ("Timed Out?"=w423:bool)  [unwired: 1 out]
          }
          frame 1 {
            n113 = xnode ("FIFO Method Node")("Element"=w425, "Timeout"=0, "FIFO In"=refnum<k21> "I2C write 1" ("FIFO")) -> ("Timed Out?"=w427:bool)  [unwired: 1 out]
          }
          frame 2 {
            n114 = xnode ("FIFO Method Node")("Element"=w429, "Timeout"=0, "FIFO In"=refnum<k21> "I2C write 2" ("FIFO")) -> ("Timed Out?"=w431:bool)  [unwired: 1 out]
          }
          frame 3, Default {
          }
        }
      }
    }
    "Local FIFO full" <- w208
    n115 = Decrement(x=w204) -> (x-1=w205:u8)
    n116 = Select(t=w205, s=w198, f=w204) -> (s? t:f=w202:u8)
    n117 = Increment(x=w180) -> (x+1=w181:u8)
    n118 = Select(t=w181, s=w178, f=w180) -> (s? t:f=w179:u8)
    n119 = Exclusive Or(1:w186, 2:w188) -> (0:w187:bool)
    "Drain count" <- w180
  }
  n120 = timed-loop "Host multiplexer" {
    timing: w32 -> [_]
    timing-out: [_] -> w31
    shift-right: [w475] -> _
    shift-left: FALSE ("Timed Out?") -> [w439]
    shift-right: [w437] -> _
    shift-left: FALSE -> [w441]
    shift-right: [w438] -> _
    shift-left: u8 0 ("Element") -> [w473]
    shift-right: [w470] -> _
    shift-left: mux_state."scan_test" ("Enum") -> [w472]
    shift-right: [w469] -> _
    shift-left: fxp<+,1,1> 0.0 ("Timeout") -> [w461]
    shift-right: [w457] -> _
    shift-left: w25 -> [w460]
    tunnel: w25 -> [w458]
    shift-right: [w436] -> _
    shift-left: u16 0 ("y") -> [w454]
    shift-right: [w446] -> _
    shift-left: u8 0 ("Element") -> [w449]
    shift-right: [w443] -> _
    shift-left: FALSE ("x = 0?") -> [w442]
    stop <- FALSE stop-if-true
    w466 = fxp<+,1,1> 0.0  # First bus
    w468 = fxp<+,2,2> 3.0  # Last bus
    # "This multiplexer is used to insert the bus and timestamp header  into the status data stream."
    n121 = Or(x=w442, y=w439) -> (x .or. y?=w440:bool)
    n122 = To Unsigned Byte Integer(number=w461) -> (unsigned 8bit integer=w462:u8)
    n123 = case shown="False" w440 {
      tunnel: [w561 w581] -> w438
      tunnel: [w560 w580] -> w437
      tunnel: w473 -> [w557 w581]
      tunnel: w461 -> [w558 _]
      tunnel: w441 -> [_ w580]
      frame False {
        n124 = case shown="0" w558 {
          tunnel: [w563 w567 w571 w575 w579] -> w561
          tunnel: [w562 w566 w570 w574 TRUE ("Timed Out?")] -> w559
          tunnel: w557 -> [_ _ _ _ w579]
          frame 0 {
            n125 = xnode ("FIFO Method Node")("Timeout"=0, "FIFO In"=refnum<k21> "I2C read 0") -> ("Element"=w563:u8, "Timed Out?"=w562:bool)  [unwired: 1 out]
          }
          frame 1 {
            n126 = xnode ("FIFO Method Node")("Timeout"=0, "FIFO In"=refnum<k21> "I2C read 1") -> ("Element"=w567:u8, "Timed Out?"=w566:bool)  [unwired: 1 out]
          }
          frame 2 {
            n127 = xnode ("FIFO Method Node")("Timeout"=0, "FIFO In"=refnum<k21> "I2C read 2") -> ("Element"=w571:u8, "Timed Out?"=w570:bool)  [unwired: 1 out]
          }
          frame 3 {
            n128 = xnode ("FIFO Method Node")("Timeout"=0, "FIFO In"=refnum<k21> "Local read") -> ("Element"=w575:u8, "Timed Out?"=w574:bool)  [unwired: 1 out]
          }
          frame 4, Default {
            # "Bad bus #, shouldn't happen."
          }
        }
        n129 = Not(x=w559) -> (.not. x?=w560:bool)
      }
      frame True {
        # "Can't read until some stuff gets written"
      }
    }
    "Mux data" <- w438
    "Mux data ready" <- w437
    n130 = case shown="\"push_TS_hi\"" w472 {
      tunnel: [w479 w492 w506 w517 w528 w540 w545] -> w463
      tunnel: [w477 w491 w504 w518 w527 w537 w548] -> w471
      tunnel: [w482 w497 w510 w522 w531 w538 w549] -> w470
      tunnel: w439 -> [_ w495 w509 w521 w530 _ w546]
      tunnel: w472 -> [w476 w494 w508 w520 w529 w536 w547]
      tunnel: [w478 w496 w506 w517 w528 w540 w550] -> w451
      tunnel: [w481 w492 w505 w519 w528 w540 w550] -> w444
      tunnel: [w481 w493 w507 w517 w528 w540 w550] -> w450
      tunnel: w437 -> [w480 _ _ _ _ w539 _]
      tunnel: [w477 w491 w504 w518 w527 w537 w548] -> w443
      frame "scan_test", Default {
        w481 = FALSE ("x = 0?")
        # "Testing whether data is ready on bus."
        n131 = case shown="True" w480 {
          tunnel: [mux_state."push_bus" ("Enum") w487] -> w482
          tunnel: [TRUE ("x = 0?") FALSE ("x = 0?")] -> w477
          tunnel: [FALSE ("x = 0?") TRUE ("x = 0?")] -> w479
          tunnel: [TRUE ("x = 0?") FALSE ("x = 0?")] -> w478
          tunnel: w476 -> [_ w487]
          frame True {
            # "Have status code in \"Data\"\nPush bus number next."
          }
          frame False {
            # "No data on bus, increment and keep waiting"
          }
        }
      }
      frame "push_bus" {
        w491 = TRUE ("x = 0?")
        w492 = FALSE ("x = 0?")
        # "Pushing bus number"
        n132 = case shown="False" w495 {
          tunnel: [w499 mux_state."push_TS_hi" ("Enum")] -> w497
          tunnel: [TRUE ("x = 0?") FALSE ("x = 0?")] -> w496
          tunnel: w494 -> [w499 _]
          tunnel: [FALSE ("x = 0?") TRUE ("x = 0?")] -> w493
          frame True {
            # "Keep trying to write."
          }
          frame False {
            # "Wrote bus number, now timestamp MSB"
          }
        }
      }
      frame "push_TS_hi" {
        w504 = TRUE ("x = 0?")
        w506 = FALSE ("x = 0?")
        # "Pushing timestamp hi byte"
        n133 = case shown="False" w509 {
          tunnel: [w513 mux_state."push_TS_lo" ("Enum")] -> w510
          tunnel: w508 -> [w513 _]
          tunnel: [TRUE ("x = 0?") FALSE ("x = 0?")] -> w507
          tunnel: [FALSE ("x = 0?") TRUE ("x = 0?")] -> w505
          frame True {
            # "Keep trying to write."
          }
          frame False {
            # "Wrote timestamp hi, now lo"
          }
        }
      }
      frame "push_TS_lo" {
        w518 = TRUE ("x = 0?")
        w517 = FALSE ("x = 0?")
        # "Pushing timestamp lo byte"
        n134 = case shown="False" w521 {
          tunnel: [w524 mux_state."copy_code" ("Enum")] -> w522
          tunnel: w520 -> [w524 _]
          tunnel: [TRUE ("x = 0?") FALSE ("x = 0?")] -> w519
          frame True {
            # "Keep trying to write."
          }
          frame False {
            # "Wrote timestamp lo, now status code\n(still in \"Data buf\")"
          }
        }
      }
      frame "copy_code" {
        w528 = FALSE ("x = 0?")
        # "Pushing status code"
        n135 = case shown="False" w530 {
          tunnel: [w533 mux_state."load_arg" ("Enum")] -> w531
          tunnel: w529 -> [w533 _]
          tunnel: [TRUE ("x = 0?") FALSE ("x = 0?")] -> w527
          frame True {
            # "Keep trying to write."
          }
          frame False {
            # "Try to read arg"
            # "Wrote  status code, now handle arg"
          }
        }
      }
      frame "load_arg" {
        w540 = FALSE ("x = 0?")
        # "Waiting for status arg to load"
        n136 = case shown="True" w539 {
          tunnel: [TRUE ("x = 0?") FALSE ("x = 0?")] -> w537
          tunnel: [mux_state."copy_arg" ("Enum") w543] -> w538
          tunnel: w536 -> [_ w543]
          frame True {
            # "Got arg, now push it."
          }
          frame False {
            # "Waiting for arg"
          }
        }
      }
      frame "copy_arg" {
        w550 = FALSE ("x = 0?")
        # "Wait for status arg push to finish"
        n137 = case shown="False" w546 {
          tunnel: [TRUE ("x = 0?") FALSE ("x = 0?")] -> w548
          tunnel: [w552 mux_state."scan_test" ("Enum")] -> w549
          tunnel: w547 -> [w552 _]
          tunnel: [FALSE ("x = 0?") TRUE ("x = 0?")] -> w545
          frame True {
            # "Waiting for arg to write"
          }
          frame False {
            # "Arg copied,increment bus and \nback to scan_test"
          }
        }
      }
    }
    "Mux state" <- w470
    "Mux Read inhibit" <- w443
    n138 = Select(t=w462, s=w451, f=w438) -> (s? t:f=w448:u8)
    n139 = Split Number(x=w454) -> (hi(x)=w453:u8, lo(x)=w452:u8)
    n140 = Select(t=w453, s=w450, f=w448) -> (s? t:f=w447:u8)
    n141 = Select(t=w452, s=w450, f=w449) -> (s? t:f=w446:u8)
    n142 = Equal?(x=w468, y=w461) -> (x = y?=w467:bool)
    n143 = Equal To 0?(x=w460) -> (x = 0?=w455:bool)
    n144 = Decrement(x=w460) -> (x-1=w459:fxp<+,10,10>)
    n145 = Select(t=w446, s=w444, f=w447) -> (s? t:f=w445:u8)
    n146 = Increment(x=w461) -> (x+1=w464:fxp<+,3,3>)
    n147 = Select(t=w458, s=w455, f=w459) -> (s? t:f=w457:fxp<+,10,10>)
    n148 = Select(t=w466, s=w467, f=w464) -> (s? t:f=w465:fxp<+,3,3>)
    n149 = case shown="True" w471 {
      tunnel: [FALSE ("Timed Out?") w586] -> w475
      tunnel: w445 -> [_ w585]
      frame False {
        # "\"Copy byte\" not asserted"
      }
      frame True {
        # "Copy byte to host"
        n150 = xnode ("FIFO Method Node")("Element"=w585, "Timeout"=0, "FIFO In"=refnum<k21> "Host read FIFO" ("FIFO")) -> ("Timed Out?"=w586:bool)  [unwired: 1 out]
      }
    }
    "Host FIFO full" <- w475
    n151 = Select(t=w465, s=w463, f=w461) -> (s? t:f=w469:fxp<+,3,3>)
    "Mux bus number" <- w469
    n152 = Increment(x=w454) -> (x+1=w456:u16)
    n153 = Select(t=w456, s=w455, f=w454) -> (s? t:f=w436:u16)
    "Timestamp" <- w436
  }
  n154 = node-c288(w13) -> ()
  n155 = node-c288(w17) -> ()
  n156 = node-c288(w4) -> ()
  n157 = node-c288(w11) -> ()
  n158 = node-c288(w31) -> ()
  n159 = node-c288(w2) -> ()
  n160 = node-c288(w38) -> ()
